vi "FCE_TS_Action_InitDebug.vi"(8 "err in":errorcluster) -> (0 "err out":errorcluster, 2 "Debug OUT":T2={"Debug AI"=[100.0, 0.0, 35.0, 0.0], "Debug DI"=[TRUE], "Debug Stream"=[1.0, 0.95, 0.0, 0.0, 50.0, 100.0, 100.0, 10.0, 50.0, 0.0, 0.0, 0.0, 0.0, 0.0, 0.0], "Debug Modbus"=[0.0, 0.0]})   [LabVIEW 2017]
uses:
  FCE_TS_FGlob_V001.llb/FCE_TS_FGlob_TDefEnum Stream Read Items.ctl
  FCE_TS_General_Libs/Kirschenhofer_Libs/KH Turck EthernetIP 17.12/KH TURCK TypeDefs FGlob.ctl
  FCE_TS_Globals_V001.llb/Globals_Settings_FCE_TS.vi
  FCE_TS_Globals_V001.llb/FCE_TS_Globals_Action.vi
panel:
  out "Debug_Modbus Names":string[](array[string])=["Gasdurchfluss_MB", "Temperatur_MB", "Alarmmeldungen_MB", "Hardwarefehler_MB"]
  in  "Debug_Modbus":sgl[](array[numeric])=[0.0, 0.0, 0.0, 0.0] format="%.2f"
  in  "Stream Read Items":T1=enum."Global State FCE1 [-]"
  out "Debug_Stream Names":string[](array[string])=["aFR_PCV_FCE1_AO [barg]", "Ap_Amb_FCE1_AI [mbara]", "CT_Si_FCE1_CV [°C]", "EI_BAT_FEC1_CAN [A]", "EI_LOAD_FEC1_AI [A]", "EI_S_FEC1_AI [A]", "EU_BAT_FEC1_CAN [V]", "EU_S_FEC1_AI [V]", "Esoc_BAT_FCE1_CAN [%]", "FC State FCE1 [-]", "Global State FCE1 [-]", "aFY_OTV_Open_Req_FCE1 [-]", "aFY_OTV_Close_Req_FCE1 [-]", "Watchdog FCE1 FCET [-]", "Shutdown_Req_FCE1 [-]", "FCSubstateStartup_FCE1 [-]", "FCSubstateShutdown_FCE1 [-]"]
  in  "Debug Stream":sgl[](array[numeric])=[1.0, 0.95, 0.0, 0.0, 50.0, 100.0, 100.0, 10.0, 50.0, 0.0, 0.0, 0.0, 0.0, 0.0, 0.0, 0.0, 0.0] format="%.2f"
  out "Debug_DI Names":string[](array[string])=["aAM_EXH_TS_On", "Adp_EXH_TS_On", "Adp_EXH_TS_Off", "HcH_TS_Warn", "HcH_TS_Alarm", "Reserve_DI_2_0_5", "Reserve_DI_2_0_6", "Reserve_DI_2_0_7"]
  out "Debug_AI Names":string[](array[string])=["Fp_HPRU_TS1", "Fp_HPRU_TS2", "Fp_So_TS", "AT_EXH_TS", "EU_DCDCi_TS", "EI_DCDC24V_TS", "EI_DIV25A_TS", "EI_DCDC12V_TS", "EI_ETC_TS", "EI_DIV40A_TS", "EI_DCDCi_TS", "EI_DCDCo_TS", "EI_BAT_TS", "EI_LOAD_TS", "Reserve_AI_4_2", "Reserve_AI_4_3", "AT_Si_TS", "AT_So_TS", "CT_Si_TS", "CT_So_TS", "Ck_CP1i_TS", "Cp_CP1i_TS", "Cp_CP1o_TS", "Cp_CP2o_TS"]
  in  "Debug_AI":sgl[](array[numeric])=[0.0, 0.0, 0.0, 0.0, 0.0, 0.0, 0.0, 0.0, 0.0, 0.0, 0.0, 0.0, 0.0, 0.0, 0.0, 0.0, 0.0, 0.0, 0.0, 0.0, 0.0, 0.0, 0.0, 0.0] format="%.2f"
  in  "Debug_DI":bool[](array[boolean])=[FALSE, FALSE, FALSE, FALSE, FALSE, FALSE, FALSE, FALSE]
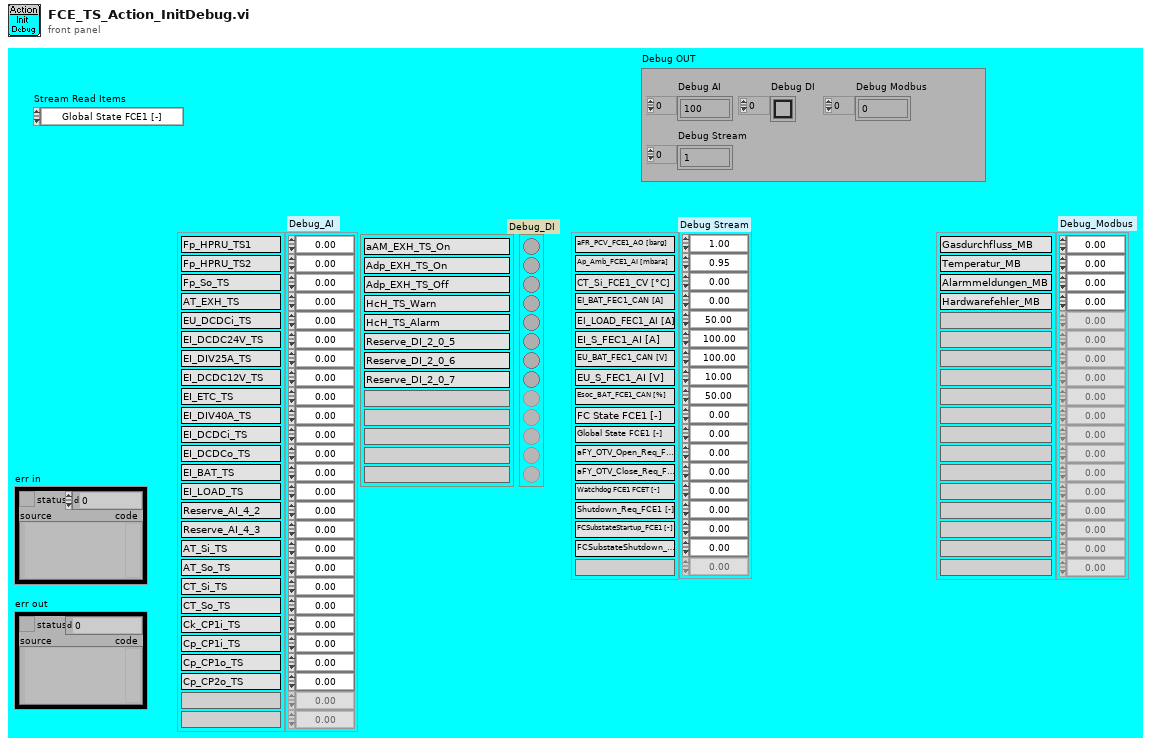
[diagram p1: front panel]
types:
  T1 = typedef "FCE_TS_FGlob_TDefEnum Stream Read Items.ctl" = enum16{"aFR_PCV_FCE1_AO [barg]", "Ap_Amb_FCE1_AI [mbara]", "CT_Si_FCE1_CV [°C]", "EI_BAT_FEC1_CAN [A]", "EI_LOAD_FEC1_AI [A]", "EI_S_FEC1_AI [A]", "EU_BAT_FEC1_CAN [V]", "EU_S_FEC1_AI [V]", "Esoc_BAT_FCE1_CAN [%]", "FC State FCE1 [-]", "Global State FCE1 [-]", "aFY_OTV_Open_Req_FCE1 [-]", "aFY_OTV_Close_Req_FCE1 [-]", "Watchdog FCE1 FCET [-]", "Shutdown_Req_FCE1 [-]", "FCSubstateStartup_FCE1 [-]", "FCSubstateShutdown_FCE1 [-]"}
  T2 = cluster{"Debug AI":sgl[], "Debug DI":bool[], "Debug Stream":sgl[], "Debug Modbus":sgl[]}
  T3 = typedef "WL_Modbus_TypeDefs_Cluster_SettingsReadReal.ctl" = cluster{"Signal Name":string[], "Description":string[], "Phys Unit":string[], "Var Type":enum16{"short", "unsigned", "float"}[], "StartAdd":u16[], "Conversion LSB":string[], "Var Size":enum16{"16 Bit", "32 Bit"}[]}
  T4 = typedef "KH_DAQ_TypeDefs_Cluster AI.ctl" = cluster{"Signal Name":string[], "Description":string[], "Phys Unit":string[], "Messbereich":T5[], "Chan":u16[], "Phys Min":sgl[], "Phys Max":sgl[], "Offset":sgl[], "Nr":u16[], "SensorType 2":T6[], "Bereich":T7[]}
  T5 = typedef "KH_DAQ_TypeDefs_Messbereich.ctl" = enum16{"-10V ... +10V", "0V ... +10V", "+2V ... +10V", "0V ... +5V", "+1V ... +5V", "-1V ... +1V", "-500mV ... +500mV", "-100mV ... +100mV", "-50mV ... +50mV", "0mA ... +20mA", "+4mA ... +20mA", "-20mA ... +20mA", "0 Ohm ... 100 Ohm", "0 Ohm ... 400 Ohm", "0 Ohm ... 2000 Ohm", "0 Ohm ... 4000 Ohm", "-200°C ... 150°C PT100", "-200°C ... 150°C PT200", "-200°C ... 150°C PT500", "-200°C ... 150°C PT1000", "-60°C ... 150°C Ni100", "-60°C ... 150°C Ni1000", "-200°C ... 850°C PT100", "-200°C ... 850°C PT200", "-200°C ... 850°C PT500", "-200°C ... 850°C PT1000", "-50°C ... 250°C Ni100", "-50°C ... 250° Ni 1000"}
  T6 = typedef "KH EthernetIPConfig TypeDefs ModuleTyp.ctl" = enum16{"TBEN-S2-4AI", "TBEN-S1-8DXP", "TBEN-S2-2RFID-4DXP", "TBEN-S2-4AO", "TBEN-S2-4IOL"}
  T7 = typedef "KH_DAQ_TypeDefs_Bereich.ctl" = enum16{"Standard", "extended Range", "NE43", ""}
  T8 = typedef "KH_DAQ_TURCK_TypeDefs_Cluster DI.ctl" = cluster{"Signal Name":string[], "Description":string[], "Chan":u16[], "Inv":bool[], "Nr":u16[], "SensorType":T6[]}
  T9 = typedef "KH TURCK TypeDefs FGlob.ctl" = enum16{"Put one", "Put all", "Recall one", "Recall all"}
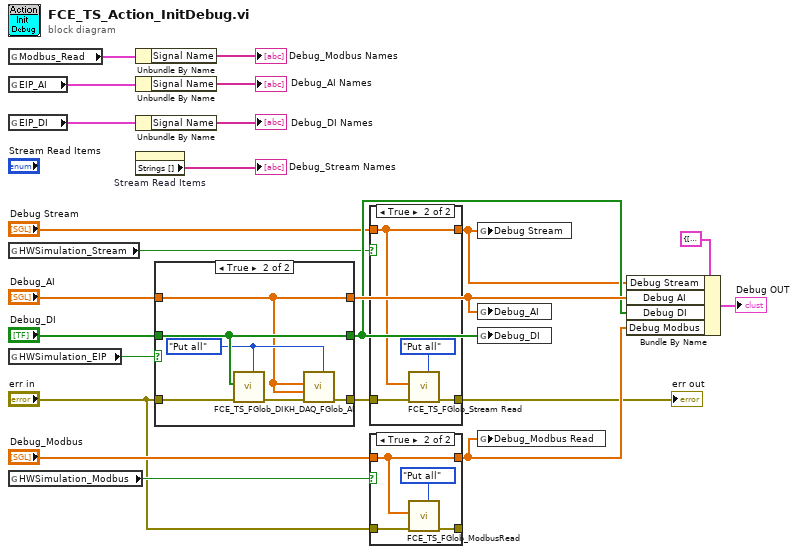
[diagram p0: block diagram]
diagram:
  n1 = global read "Globals_Settings_FCE_TS.vi" "Modbus_Read"() -> (w4:T3)
  n2 = global read "Globals_Settings_FCE_TS.vi" "EIP_AI"() -> (w23:T4)
  n3 = global read "Globals_Settings_FCE_TS.vi" "EIP_DI"() -> (w22:T8)
  n4 = global read "Globals_Settings_FCE_TS.vi" "HWSimulation_Stream"() -> (w13:bool)
  n5 = global read "Globals_Settings_FCE_TS.vi" "HWSimulation_EIP"() -> (w20:bool)
  n6 = global read "Globals_Settings_FCE_TS.vi" "HWSimulation_Modbus"() -> (w7:bool)
  n7 = Unbundle By Name(w4) -> ("Signal Name"=→"Debug_Modbus Names":string[])
  n8 = Unbundle By Name(w23) -> ("Signal Name"=→"Debug_AI Names":string[])
  n9 = Unbundle By Name(w22) -> ("Signal Name"=→"Debug_DI Names":string[])
  n10 = property on="Stream Read Items" class="Enum (strict)"() -> ("Strings []"=→"Debug_Stream Names":string[])  [unwired: 2 in, 2 out]
  n11 = case shown="True" w20 {
    tunnel: "err in" -> [w26 w30]
    tunnel: [w26 w28] -> w12
    tunnel: "Debug_DI" -> [w24 w31]
    tunnel: "Debug_AI" -> [w25 w27]
    tunnel: [w25 w27] -> w16
    tunnel: [w24 w31] -> w15
    frame False {
    }
    frame True {
      w29 = KH_TURCK_TypeDefs_FGlob."Put all" ("Function (Recall One)")
      n12 = call "FCE_TS_FGlob_DI.vi"("Function (Recall One)"=w29, "err in"=w30, "DI Values IN"=w31) -> ("err out"=w32:errorcluster)  [unwired: 6 in, 2 out]
      n13 = call "KH_DAQ_FGlob_AI.vi"("Function (Recall One)"=w29, "err in"=w32, "AI Unscaled IN"=w27, "AI Values IN"=w27) -> ("err out"=w28:errorcluster)  [unwired: 4 in, 3 out]
    }
  }
  n14 = case shown="True" w13 {
    tunnel: w12 -> [w34 w38]
    tunnel: "Debug Stream" -> [w33 w35]
    tunnel: [w34 w36] -> w1
    tunnel: [w33 w35] -> w10
    frame False {
    }
    frame True {
      n15 = call "FCE_TS_FGlob_Stream Read.vi"("Function (Recall One)"=KH_TURCK_TypeDefs_FGlob."Put all", "err in"=w38, "AI Values IN"=w35) -> ("err out"=w36:errorcluster)  [unwired: 6 in, 2 out]
    }
  }
  "err out" <- w1
  n16 = case shown="True" w7 {
    tunnel: "err in" -> [w40 w44]
    tunnel: "Debug_Modbus" -> [w39 w42]
    tunnel: [w40 w43] -> _
    tunnel: [w39 w42] -> w2
    frame False {
    }
    frame True {
      n17 = call "FCE_TS_FGlob_ModbusRead.vi"("Function (Recall One)"=KH_TURCK_TypeDefs_FGlob."Put all", "err in"=w44, "AI Values IN"=w42) -> ("err out"=w43:errorcluster)  [unwired: 6 in, 2 out]
    }
  }
  n18 = global write "FCE_TS_Globals_Action.vi" "Debug Stream"(w10) -> ()
  n19 = global write "FCE_TS_Globals_Action.vi" "Debug_AI"(w16) -> ()
  n20 = global write "FCE_TS_Globals_Action.vi" "Debug_DI"(w15) -> ()
  n21 = global write "FCE_TS_Globals_Action.vi" "Debug_Modbus Read"(w2) -> ()
  n22 = Bundle By Name(cluster=T2 {"Debug AI"=[], "Debug DI"=[], "Debug Stream"=[], "Debug Modbus"=[]} ("Debug OUT"), "Debug Stream"=w10, "Debug AI"=w16, "Debug DI"=w15, "Debug Modbus"=w2) -> (→"Debug OUT":T2)
